vi "WPI_DisableFilter.vi"(8 "error in (no error)":errorcluster, 11 "DigitalInputDevRef":T1={"DevStatus"={"status"=FALSE, "code"=0, "source"=""}, "DIO Channel"=enum."DIO 1"}) -> (0 "error out":errorcluster, 3 "DigitalInputDevRef":T1={"DevStatus"={"status"=FALSE, "code"=0, "source"=""}, "DIO Channel"=enum."DIO 1"})   [LabVIEW 2017]
doc: "Disables the digital input filter you enable with the SetFilterFrequency VI.\n\nThis software is licensed. Open the labview\\readme\\WPI Robotics Library Open Source License.txt file for more information."
uses:
  <vilib>/Rock Robotics/WPI/DigitalInput/WPI_DigitalInputDevRef.ctl
  <vilib>/Rock Robotics/SystemInterfaces/DIO/FPGA_DIOChannel.ctl
  <vilib>/Rock Robotics/SystemInterfaces/System/FPGA_SystemGet.vi
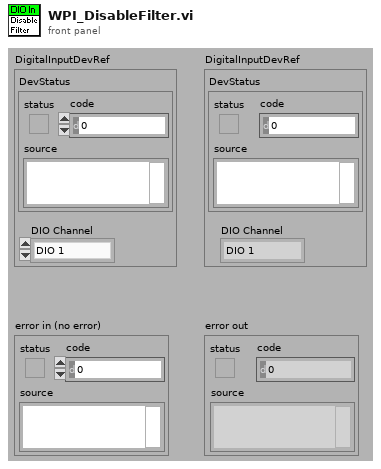
[diagram p1: front panel]
types:
  T1 = typedef "WPI_DigitalInputDevRef.ctl" = cluster{"DevStatus":errorcluster, "DIO Channel":T2}
  T2 = typedef "FPGA_DIOChannel.ctl" = enum8{"DIO 0", "DIO 1", "DIO 2", "DIO 3", "DIO 4", "DIO 5", "DIO 6", "DIO 7", "DIO 8", "DIO 9", "DIO MXP 0", "DIO MXP 1", "DIO MXP 2", "DIO MXP 3", "DIO MXP 4", "DIO MXP 5", "DIO MXP 6", "DIO MXP 7", "DIO MXP 8", "DIO MXP 9", "DIO MXP 10", "DIO MXP 11", "DIO MXP 12", "DIO MXP 13", "DIO MXP 14", "DIO MXP 15", "SPI Port CS1", "SPI Port CS2", "SPI Port CS3", "SPI Port MISO", "SPI Port MOSI", "Invalid"}
  T3 = typedef "FPGA_DIODevRef.ctl" = cluster{"DevStatus":errorcluster}
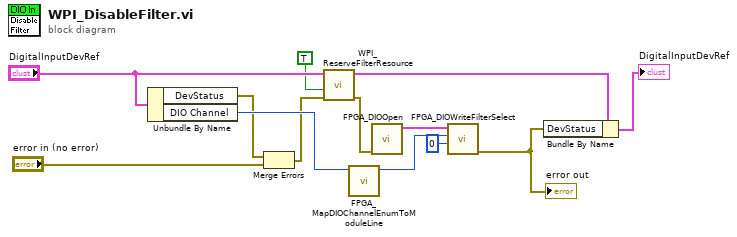
[diagram p0: block diagram]
diagram:
  n1 = Unbundle By Name("DigitalInputDevRef") -> ("DevStatus"=w2:errorcluster, "DIO Channel"=w6:T2)
  n2 = Merge Errors(w2, "error in (no error)") -> (w1:errorcluster)
  n3 = call <vilib>:"WPI_ReserveFilterResource.vi"("error in (no error)"=w1, "Release Filter"=TRUE, "DigitalInputDevRef"="DigitalInputDevRef") -> ("error out"=w8:errorcluster, "DigitalInputDevRef"=w11:T1)  [unwired: 1 in, 6 out]
  n4 = call <vilib>:"FPGA_MapDIOChannelEnumToModuleLine.vi"("DIOChannel"=w6) -> ("ActualDIOChannel(U8)"=w5:u8)  [unwired: 10 out]
  n5 = call <vilib>:"FPGA_DIOOpen.vi"("error in (no error)"=w8) -> ("DIODeviceRef"=w7:T3)  [unwired: 1 in, 9 out]
  n6 = call <vilib>:"FPGA_DIOWriteFilterSelect.vi"("PWMFilterSelect"=u8 0, "channel index"=w5, "DIODeviceRef"=w7) -> ("error out"=w12:errorcluster)  [unwired: 1 in, 7 out]
  "error out" <- w12
  n7 = Bundle By Name(cluster=w11, "DevStatus"=w12) -> (→"DigitalInputDevRef":T1)
